vi "GeraeteKennung aus GeraeteType.vi"(8 "error in (no error)":errorcluster caption="Fehler (Eingang, kein Fehler)", 10 "Gerätetype":string, 11 "Steuerung PNS Eingang":refnum<class "Steuerung PNS.lvclass">) -> (0 "error out":errorcluster caption="Fehler (Ausgang)", 2 "Gerätekennung":i32, 3 "Steuerung PNS Ausgang":refnum<class "Steuerung PNS.lvclass">)   [LabVIEW 2015, in "Steuerung PNS.lvclass"]
uses:
  Steuerung PNS.lvclass
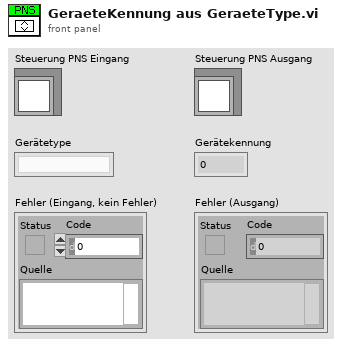
[diagram p1: front panel]
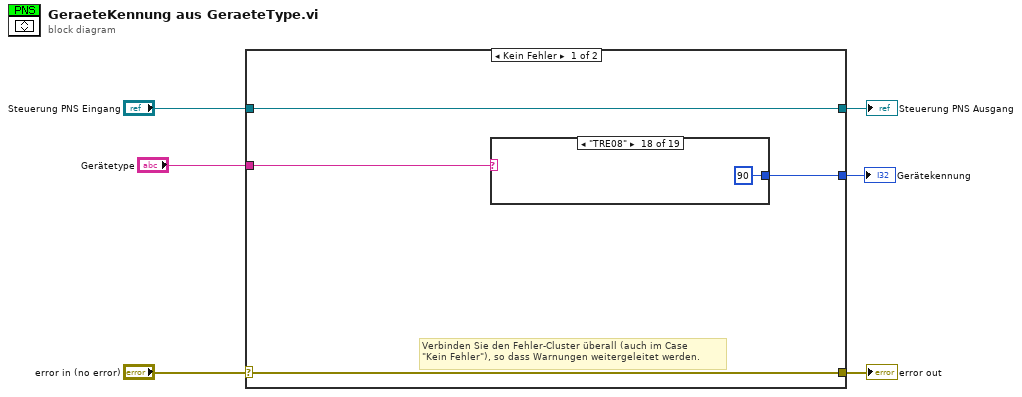
[diagram p0: block diagram]
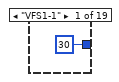
[diagram p2: hidden frame]
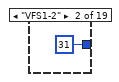
[diagram p3: hidden frame]
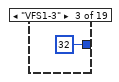
[diagram p4: hidden frame]
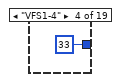
[diagram p5: hidden frame]
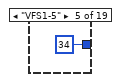
[diagram p6: hidden frame]
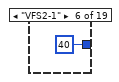
[diagram p7: hidden frame]
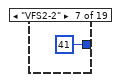
[diagram p8: hidden frame]
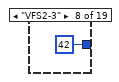
[diagram p9: hidden frame]
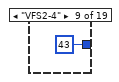
[diagram p10: hidden frame]
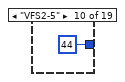
[diagram p11: hidden frame]
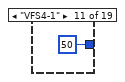
[diagram p12: hidden frame]
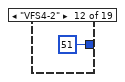
[diagram p13: hidden frame]
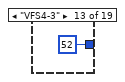
[diagram p14: hidden frame]
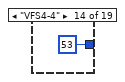
[diagram p15: hidden frame]
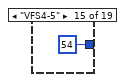
[diagram p16: hidden frame]
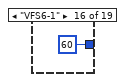
[diagram p17: hidden frame]
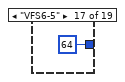
[diagram p18: hidden frame]
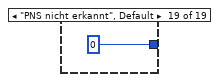
[diagram p19: hidden frame]
diagram:
  n1 = case shown="Kein Fehler" "error in (no error)" {
    selector: "error in (no error)" -> [w9 w31]
    tunnel: [w9 w31] -> w5
    tunnel: [w10 w30] -> w3
    tunnel: "Steuerung PNS Eingang" -> [w10 w30]
    tunnel: "Gerätetype" -> [w8 _]
    tunnel: [w7 _] -> w1
    frame No Error {
      # "Verbinden Sie den Fehler-Cluster überall (auch im Case\n\"Kein Fehler\"), so dass Warnungen weitergeleitet werden."
      n2 = case shown="\"TRE08\"" w8 {
        tunnel: [30 31 32 33 34 40 41 42 43 44 50 51 52 53 54 60 64 90 0] -> w7
        frame "VFS1-1" {
        }
        frame "VFS1-2" {
        }
        frame "VFS1-3" {
        }
        frame "VFS1-4" {
        }
        frame "VFS1-5" {
        }
        frame "VFS2-1" {
        }
        frame "VFS2-2" {
        }
        frame "VFS2-3" {
        }
        frame "VFS2-4" {
        }
        frame "VFS2-5" {
        }
        frame "VFS4-1" {
        }
        frame "VFS4-2" {
        }
        frame "VFS4-3" {
        }
        frame "VFS4-4" {
        }
        frame "VFS4-5" {
        }
        frame "VFS6-1" {
        }
        frame "VFS6-5" {
        }
        frame "TRE08" {
        }
        frame "PNS nicht erkannt", Default {
        }
      }
    }
    frame Error {
    }
  }
  "error out" <- w5
  "Steuerung PNS Ausgang" <- w3
  "Gerätekennung" <- w1
